vi "Teleop.vi"(10 "Match Info":T1={"Autonomous Elapsed Seconds"=0.0, "TeleOp Elapsed Seconds"=0.0, "Disabled Elapsed Seconds"=0.0, "Visited Autonomous"=FALSE, "Visited TeleOp"=FALSE, "Visited Disabled"=FALSE, "Autonomous Settings"={"Autonomous Style"=enum."Independent", "VI Refnum"=refnum}}, 11 "Call Context":T2) -> ()   [LabVIEW 2013]
doc: "This VI is called for each TeleOp packet received from the DS where the robot is not disabled. It is often used to read from the joysticks and update I/O or to update setpoints for timed control loops. It should complete and return within 20 milliseconds or it may miss DS packets."
uses:
  <vilib>/Rock Robotics/WPI/DriverStation/WPI_DriverStationDerivedRobotMode.ctl
  <vilib>/Rock Robotics/WPI/DriverStation/WPI_DriverStationMatch Info.ctl
  <vilib>/Rock Robotics/WPI/Solenoid/WPI_SolenoidValue.ctl
  Robot Global Data.vi
  <vilib>/Rock Robotics/WPI/Solenoid/WPI_SolenoidSetEnum.vi
  <vilib>/Rock Robotics/WPI/Joystick/WPI_JoystickGetSetRefNum.vi
  <vilib>/Rock Robotics/WPI/RobotDrive/WPI_RobotDriveGetSetRefNum.vi
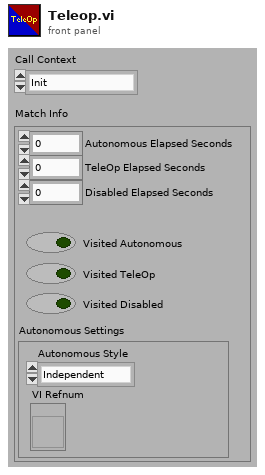
[diagram p1: front panel]
types:
  T1 = typedef "WPI_DriverStationMatch Info.ctl" = cluster{"Autonomous Elapsed Seconds":dbl, "TeleOp Elapsed Seconds":dbl, "Disabled Elapsed Seconds":dbl, "Visited Autonomous":bool, "Visited TeleOp":bool, "Visited Disabled":bool, "Autonomous Settings":cluster{"Autonomous Style":enum16{"Iterative", "Independent"}, "VI Refnum":refnum<vi>}}
  T2 = typedef "WPI_DriverStationDerivedRobotMode.ctl" = enum16{"Init", "Execute", "Stop"}
  T3 = typedef "WPI_SolenoidValue.ctl" = enum16{"Off", "On", "Forward", "Reverse"}
  T4 = typedef "WPI_JoystickDevRef.ctl" = cluster{"Device":T5}
  T5 = typedef "WPI_JoystickDeviceEnum.ctl" = enum16{"USB 1", "USB 2", "USB 3", "USB 4", "Kinect 1", "Kinect 2"}
  T6 = cluster{"A":bool, "B":bool, "X":bool, "Y":bool, "LB":bool, "RB":bool, "Back":bool, "Start":bool, "LS":bool, "RS":bool}
  T7 = cluster{"Left Stick (x)":dbl, "Left Stick (y)":dbl, "Trigger Axis":dbl, "Right Stick (x)":dbl, "Right Stick (y)":dbl}
  T8 = typedef "WPI_RobotDriveDevRef.ctl" = cluster{"DevStatus":errorcluster, "Motors[]":T9[], "Square Inputs":bool, "Max Output":dbl, "Isochronous":bool}
  T9 = typedef "WPI_MotorControlDeviceRef.ctl" = cluster{"DeviceStatus":errorcluster, "Type":enum16{"PWM", "CAN"}, "PWM":cluster{"Digital Module":T10, "PWM Channel":T11, "DeadBand":T12}, "CAN":cluster{"Device Number":u8, "Control Mode":T13, "Semaphore":T14, "Max Vout":dbl}, "Invert":bool, "TransformRef":T15, "InvTransformRef":T15}
  T10 = typedef "FPGA_TypedefDigitalModule.ctl" = enum16{"Digital Module 1", "Digital Module 2"}
  T11 = typedef "FPGA_DIOPWMChannel.ctl" = enum8{"PWM 1", "PWM 2", "PWM 3", "PWM 4", "PWM 5", "PWM 6", "PWM 7", "PWM 8", "PWM 9", "PWM 10", "Invalid"}
  T12 = typedef "WPI_PWMDeadband.ctl" = cluster{"Name":string, "maxPositivePwm":i32, "minPositivePwm":i32, "centerPwm":i32, "maxNegativePwm":i32, "minNegativePwm":i32, "angularRange":u16}
  T13 = typedef "WPI_CANJaguar_ControlMode.ctl" = enum8{"Percent VBus", "Current", "Speed", "Position", "Voltage"}
  T14 = typedef "Semaphore RefNum" = refnum<k1>
  T15 = typedef "WPI_PWMTransform_ConPane.ctl" = refnum<vi>
  T16 = typedef "WPI_JoystickButtonState.ctl" = cluster{"Button 1":bool, "Button 2":bool, "Button 3":bool, "Button 4":bool, "Button 5":bool, "Button 6":bool, "Button 7":bool, "Button 8":bool, "Button 9":bool, "Button 10":bool, "Button 11":bool, "Button 12":bool}
  T17 = cluster{"axis 1 (x)":dbl, "axis 2 (y)":dbl, "axis 3 (throttle)":dbl, "axis 4":dbl, "axis 5":dbl, "axis 6":dbl}
  T18 = typedef "WPI_DigitalInputDevRef.ctl" = cluster{"DevStatus":errorcluster, "DIO Channel":T19, "Digital Module":T10}
  T19 = typedef "FPGA_DIOChannel.ctl" = enum8{"DIO 1", "DIO 2", "DIO 3", "DIO 4", "DIO 5", "DIO 6", "DIO 7", "DIO 8", "DIO 9", "DIO 10", "DIO 11", "DIO 12", "DIO 13", "DIO 14", "Invalid"}
  T20 = typedef "WPI_SolenoidDevRef.ctl" = cluster{"DevStatus":errorcluster, "Solenoid Module":T21, "Forward Solenoid Channel":T22, "Reverse Solenoid Channel":T22}
  T21 = typedef "FPGA_TypedefSolenoidModule.ctl" = enum16{"Solenoid Module 1", "Solenoid Module 2"}
  T22 = typedef "WPI_SolenoidChannel.ctl" = enum8{"Solenoid 1", "Solenoid 2", "Solenoid 3", "Solenoid 4", "Solenoid 5", "Solenoid 6", "Solenoid 7", "Solenoid 8", "Invalid"}
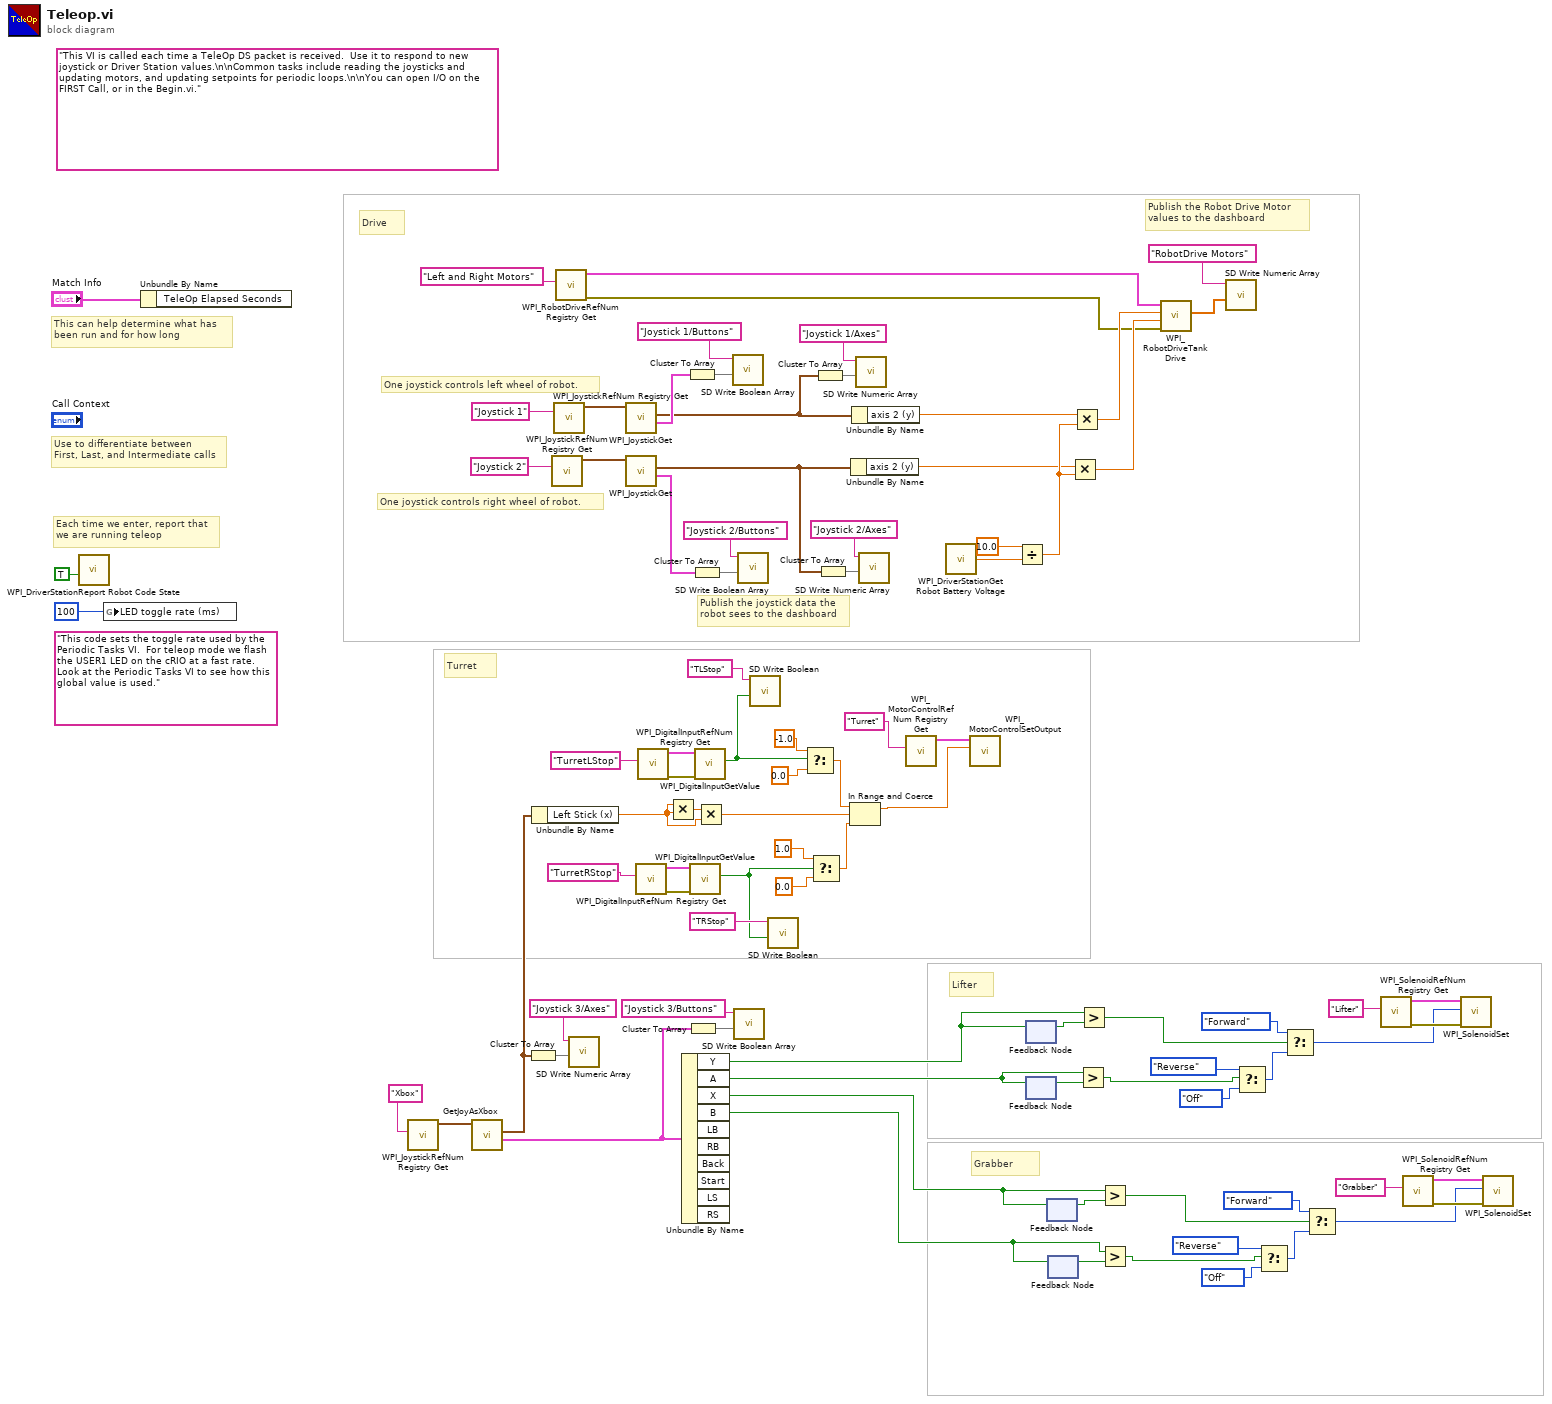
[diagram p0: block diagram]
diagram:
  (unwired) "This code sets the toggle rate used by the Periodic Tasks VI.  For teleop mode we flash the USER1 LED on the cRIO at a fast rate.  Look at the Periodic Tasks VI to see how this global value is used."
  (unwired) "This VI is called each time a TeleOp DS packet is received.  Use it to respond to new joystick or Driver Station values.\n\nCommon tasks include reading the joysticks and updating motors, and updating setpoints for periodic loops.\n\nYou can open I/O on the FIRST Call, or in the Begin.vi."
  # "Grabber"
  # "Lifter"
  # "Turret"
  # "Drive"
  # "Publish the joystick data the\nrobot sees to the dashboard"
  # "Publish the Robot Drive Motor\nvalues to the dashboard"
  # "One joystick controls right wheel of robot."
  # "One joystick controls left wheel of robot."
  # "Each time we enter, report that\nwe are running teleop"
  # "Use to differentiate between\nFirst, Last, and Intermediate calls"
  # "This can help determine what has\nbeen run and for how long"
  n1 = call <vilib>:"WPI_DriverStationReport Robot Code State.vi"("TeleOp"=TRUE ("Autonomous")) -> ()  [unwired: 10 in, 1 out]
  n2 = global write "Robot Global Data.vi" "LED toggle rate (ms)"(u32 100 ("LED ms toggle rate")) -> ()
  n3 = Unbundle By Name("Match Info") -> ()  [unwired: 1 out]
  n4 = call <vilib>:"WPI_JoystickRefNum Registry Get.vi"("refnum name"="Xbox") -> ("JoystickDevRef"=w65:T4)  [unwired: 9 in, 1 out]
  n5 = call "GetJoyAsXbox.vi"("JoystickDevRef"=w65) -> ("Buttons"=w53:T6, "Axes"=w50:T7)  [unwired: 8 in, 1 out]
  n6 = Cluster To Array(cluster=w50) -> (array=w52:dbl[])
  n7 = Unbundle By Name(w50) -> ("Left Stick (x)"=w30:dbl)
  n8 = call <vilib>:"WPI_JoystickRefNum Registry Get.vi"("refnum name"="Joystick 2") -> ("JoystickDevRef"=w83:T4)  [unwired: 9 in, 1 out]
  n9 = call <vilib>:"WPI_JoystickRefNum Registry Get.vi"("refnum name"="Joystick 1") -> ("JoystickDevRef"=w85:T4)  [unwired: 9 in, 1 out]
  n10 = call <vilib>:"WPI_RobotDriveRefNum Registry Get.vi"("refnum name"="Left and Right Motors") -> ("error out"=w42:errorcluster, "RobotDriveDevRef"=w67:T8)  [unwired: 9 in]
  n11 = call <vilib>:"SD Write Numeric Array.vi"("Numeric Array"=w52, "Name"="Joystick 3/Axes") -> ()  [unwired: 8 in, 2 out]
  n12 = call <vilib>:"WPI_JoystickGet.vi"("JoystickDevRef"=w85) -> ("Buttons"=w71:T16, "Axes"=w70:T17)  [unwired: 4 in, 1 out]
  n13 = call <vilib>:"WPI_JoystickGet.vi"("JoystickDevRef"=w83) -> ("Buttons"=w72:T16, "Axes"=w73:T17)  [unwired: 4 in, 1 out]
  n14 = call <vilib>:"WPI_DigitalInputRefNum Registry Get.vi"("refnum name"="TurretRStop") -> ("error out"=w59:errorcluster, "DigitalInputDevRef"=w58:T18)  [unwired: 9 in]
  n15 = call <vilib>:"WPI_DigitalInputRefNum Registry Get.vi"("refnum name"="TurretLStop") -> ("error out"=w62:errorcluster, "DigitalInputDevRef"=w61:T18)  [unwired: 9 in]
  n16 = Multiply(x=w30, y=w30) -> (x*y=w31:dbl)
  n17 = Unbundle By Name(w53) -> ("Y"=w24:bool, "A"=w21:bool, "X"=w2:bool, "B"=w1:bool)  [unwired: 6 out]
  n18 = Cluster To Array(cluster=w71) -> (array=w81:bool[])
  n19 = Cluster To Array(cluster=w53) -> (array=w55:bool[])
  n20 = call <vilib>:"WPI_DigitalInputGetValue.vi"("error in (no error)"=w59, "DigitalInputDevRef"=w58) -> ("Value"=w40:bool)  [unwired: 7 in, 2 out]
  n21 = Cluster To Array(cluster=w72) -> (array=w77:bool[])
  n22 = call <vilib>:"WPI_DigitalInputGetValue.vi"("error in (no error)"=w62, "DigitalInputDevRef"=w61) -> ("Value"=w41:bool)  [unwired: 7 in, 2 out]
  n23 = Multiply(x=w31, y=w30) -> (x*y=w29:dbl)
  n24 = call <vilib>:"SD Write Boolean Array.vi"("Boolean Array"=w81, "Name"="Joystick 1/Buttons") -> ()  [unwired: 8 in, 2 out]
  n25 = call <vilib>:"SD Write Boolean Array.vi"("Boolean Array"=w55, "Name"="Joystick 3/Buttons") -> ()  [unwired: 8 in, 2 out]
  n26 = call <vilib>:"SD Write Boolean Array.vi"("Boolean Array"=w77, "Name"="Joystick 2/Buttons") -> ()  [unwired: 8 in, 2 out]
  n27 = call <vilib>:"SD Write Boolean.vi"("Boolean"=w41, "Name"="TLStop") -> ()  [unwired: 8 in, 2 out]
  n28 = call <vilib>:"SD Write Boolean.vi"("Boolean"=w40, "Name"="TRStop") -> ()  [unwired: 8 in, 2 out]
  n29 = Select(t=-1.0, s=w41, f=0.0) -> (s? t:f=w39:dbl)
  n30 = Select(t=1.0, s=w40, f=0.0) -> (s? t:f=w38:dbl)
  n31 = Cluster To Array(cluster=w70) -> (array=w79:dbl[])
  n32 = Cluster To Array(cluster=w73) -> (array=w75:dbl[])
  n33 = In Range and Coerce(upper limit=w39, x=w29, lower limit=w38) -> (coerced(x)=w37:dbl)  [unwired: 1 out]
  n34 = Unbundle By Name(w73) -> ("axis 2 (y)"=w46:dbl)
  n35 = Unbundle By Name(w70) -> ("axis 2 (y)"=w45:dbl)
  n36 = call <vilib>:"SD Write Numeric Array.vi"("Numeric Array"=w79, "Name"="Joystick 1/Axes") -> ()  [unwired: 8 in, 2 out]
  n37 = call <vilib>:"SD Write Numeric Array.vi"("Numeric Array"=w75, "Name"="Joystick 2/Axes") -> ()  [unwired: 8 in, 2 out]
  n38 = call <vilib>:"WPI_MotorControlRefNum Registry Get.vi"("refnum name"="Turret") -> ("MotorControlDevRef"=w36:T9)  [unwired: 9 in, 1 out]
  n39 = call <vilib>:"WPI_DriverStationGet Robot Battery Voltage.vi"() -> ("robot battery voltage"=w49:dbl)  [unwired: 14 in, 1 out]
  n40 = call <vilib>:"WPI_MotorControlSetOutput.vi"("Output"=w37, "MotorControlDevRef"=w36) -> ()  [unwired: 7 in, 3 out]
  n41 = Divide(x=10.0, y=w49) -> (x/y=w47:dbl)
  n42 = feedback-in #1(w24) -> ()
  n43 = feedback #1() -> (w23:bool)  [unwired: 1 in]
  n44 = feedback #2() -> (w22:bool)  [unwired: 1 in]
  n45 = feedback-in #2(w21) -> ()
  n46 = feedback #3() -> (w10:bool)  [unwired: 1 in]
  n47 = feedback-in #3(w2) -> ()
  n48 = feedback #4() -> (w9:bool)  [unwired: 1 in]
  n49 = feedback-in #4(w1) -> ()
  n50 = Multiply(x=w46, y=w47) -> (x*y=w44:dbl)
  n51 = Multiply(x=w45, y=w47) -> (x*y=w43:dbl)
  n52 = Greater?(x=w21, y=w22) -> (0:w19:bool)
  n53 = Greater?(x=w24, y=w23) -> (0:w20:bool)
  n54 = Greater?(x=w2, y=w10) -> (0:w8:bool)
  n55 = Greater?(x=w1, y=w9) -> (0:w7:bool)
  n56 = call <vilib>:"WPI_RobotDriveTankDrive.vi"("error in (no error)"=w42, "Right axis value"=w44, "Left axis value"=w43, "RobotDriveDevRef"=w67) -> ("Motor Values"=w69:dbl[])  [unwired: 7 out]
  n57 = call <vilib>:"SD Write Numeric Array.vi"("Numeric Array"=w69, "Name"="RobotDrive Motors") -> ()  [unwired: 8 in, 2 out]
  n58 = Select(t=WPI_SolenoidValue."Reverse" ("Value"), s=w19, f=WPI_SolenoidValue."Off" ("Value")) -> (s? t:f=w28:T3)
  n59 = Select(t=WPI_SolenoidValue."Reverse" ("Value"), s=w7, f=WPI_SolenoidValue."Off" ("Value")) -> (s? t:f=w14:T3)
  n60 = Select(t=WPI_SolenoidValue."Forward" ("Value"), s=w20, f=w28) -> (s? t:f=w15:T3)
  n61 = Select(t=WPI_SolenoidValue."Forward" ("Value"), s=w8, f=w14) -> (s? t:f=w3:T3)
  n62 = call <vilib>:"WPI_SolenoidRefNum Registry Get.vi"("refnum name"="Lifter") -> ("error out"=w17:errorcluster, "SolenoidDevRef"=w16:T20)  [unwired: 9 in]
  n63 = call <vilib>:"WPI_SolenoidRefNum Registry Get.vi"("refnum name"="Grabber") -> ("error out"=w5:errorcluster, "SolenoidDevRef"=w4:T20)  [unwired: 9 in]
  n64 = call-poly <vilib>:"WPI_SolenoidSet.vi"("error in (no error)"=w17, "Value"=w15, "SolenoidDevRef"=w16) -> ()  [unwired: 7 in, 2 out]
  n65 = call-poly <vilib>:"WPI_SolenoidSet.vi"("error in (no error)"=w5, "Value"=w3, "SolenoidDevRef"=w4) -> ()  [unwired: 7 in, 2 out]
